vi "Go to Running.vi"(8 "error in (no error)":errorcluster, 11 "Process State in":refnum<class "Process State.lvclass">) -> (0 "error out":errorcluster, 3 "Process State out":refnum<class "State Actor.lvclass">)   [LabVIEW 2025, in "Process States.lvlib" / "Process State.lvclass"]
doc: "This method defines the transition from any state to the Running state."
uses:
  Process State.lvclass
  <vilib>/ni/Actors/State Actor/State Actor/State Actor.lvclass
  Running/Running.lvclass
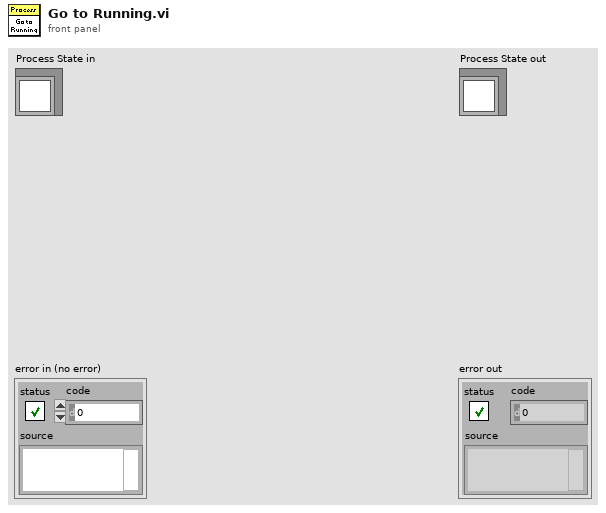
[diagram p1: front panel]
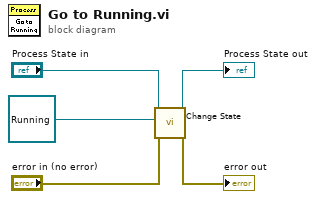
[diagram p0: block diagram]
diagram:
  n1 = call <vilib>:"Change State.vi"("error in (no error)"="error in (no error)", "New State in"=refnum<class "Running.lvclass"> refnum ("Process States.lvlib:Running.lvclass"), "State in"="Process State in") -> ("error out"=→"error out":errorcluster, "State out"=→"Process State out":refnum<class "State Actor.lvclass">)  [unwired: 7 in]
